vi "Zero Padder.vi"   [LabVIEW 2014, in "NI_AALPro.lvlib"]
doc: "Resizes the input sequence <B>Input Array</B> to the next higher valid power of 2, sets the new trailing elements of the sequence to zero, and leaves the first n elements unchanged, where n is the number of samples in the input sequence. Wire data to the <B>Input Array</B> input to determine the polymorphic instance to use or manually select the instance."
uses:
  NI_AALPro.lvlib
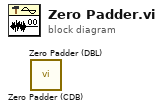
[diagram p0: block diagram]
diagram:
  n1 = call "Zero Padder (CDB).vi"() -> ()  [unwired: 11 in, 1 out]
  n2 = call "Zero Padder (DBL).vi"() -> ()  [unwired: 11 in, 1 out]
